vi "From String.vi"(8 "error in (no error)":errorcluster, 9 "initial scan location":u32, 10 "String":string, 11 "Double Float in":refnum<class "Abs_Single Float 1D.lvclass">) -> (0 "error out":errorcluster, 1 "offset past scan":u32, 2 "Remaining String":string, 3 "Double Float out":refnum<class "Abs_Single Float 1D.lvclass">)   [LabVIEW 2021, in "Abs_Single Float 1D.lvclass"]
uses:
  Abs_Single Float 1D.lvclass
  C:/TSA/LV_Abstract/Source/Abs_Types/Numeric 1D/Abs_Numeric_1D.lvclass
  Support/Type.ctl
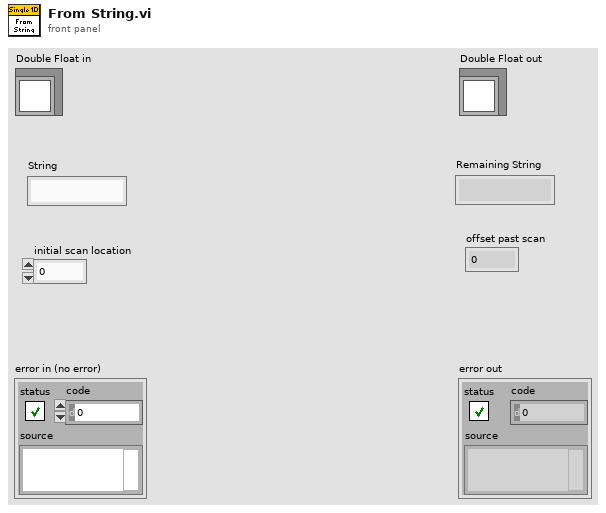
[diagram p1: front panel]
types:
  T1 = typedef "Abs_Single Float 1D.lvclass/Type.ctl" = sgl[]
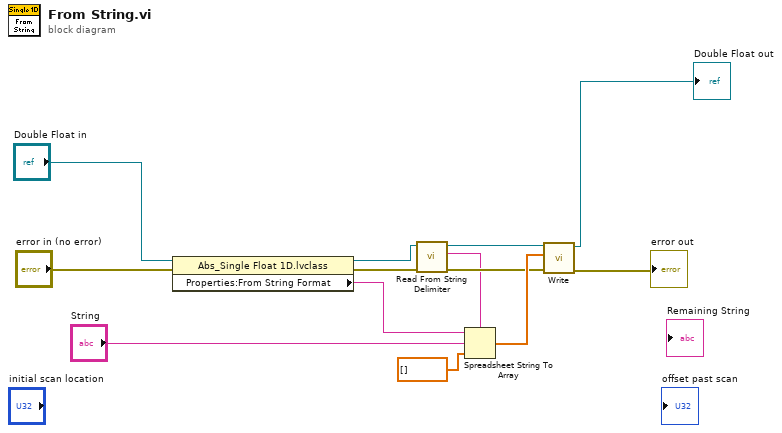
[diagram p0: block diagram]
diagram:
  n1 = property class="Abs_Single Float 1D.lvclass"(reference="Double Float in", error in="error in (no error)") -> (reference out=w2:refnum<class "Abs_Single Float 1D.lvclass">, error out=w5:errorcluster, "Properties:From String Format"=w8:string)
  n2 = call-dynamic "Read From String Delimiter.vi"("error in (no error)"=w5, "Abs_Array in"=w2) -> ("error out"=w4:errorcluster, "From String Delimiter"=w3:string, "Abs_Array out"=w1:refnum<class "Abs_Single Float 1D.lvclass">)  [unwired: 7 in]
  n3 = Spreadsheet String To Array(delimiter (Tab)=w3, format string=w8, spreadsheet string="String", array type (2D Dbl)=T1 [] ("default value 1")) -> (array=w7:sgl[])
  n4 = call-dynamic "Write.vi"("error in (no error)"=w4, "Value"=w7, "Double Float.lvclass in"=w1) -> ("error out"=→"error out":errorcluster, "Double Float.lvclass out"=→"Double Float out":refnum<class "Abs_Single Float 1D.lvclass">)  [unwired: 7 in]
